vi "Read Unfiltered Debug Data.vi"(8 "error in (no error)":errorcluster, 11 "Debugger In":refnum<class "Debugger.lvclass">) -> (0 "error out":errorcluster, 2 "Data Log":refnum<class "Debug Data.lvclass">[](array[class]), 3 "Debugger Out":refnum<class "Debugger.lvclass">)   [LabVIEW 2020, in "Debugger.lvclass"]
uses:
  Debugger.lvclass
  Debug Data/Debug Data.lvclass
  Debug Log/Debug Log.lvclass/Debug Log.ctl
  Debugger.lvclass/Debugger.ctl
  Debug Log/Debug Log.lvclass
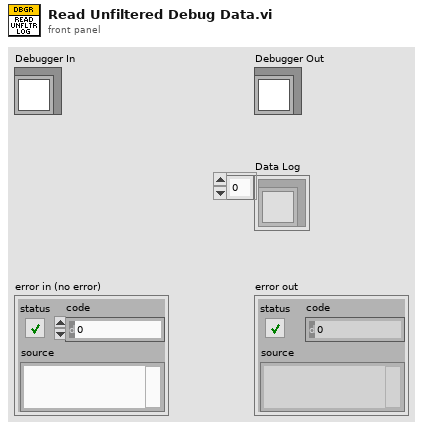
[diagram p1: front panel]
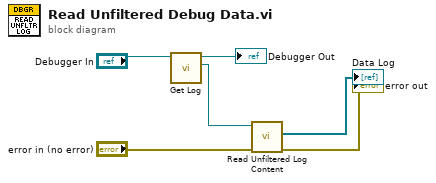
[diagram p0: block diagram]
diagram:
  n1 = call "Get Log.vi"("Debugger in"="Debugger In") -> ("Log"=w1:refnum<class "Debug Log.lvclass">, "Debugger out"=→"Debugger Out":refnum<class "Debugger.lvclass">)  [unwired: 8 in, 1 out]
  n2 = call "Read Unfiltered Log Content.vi"("error in (no error)"="error in (no error)", "Debug Log In"=w1) -> ("error out"=→"error out":errorcluster, "Data Log"=→"Data Log":refnum<class "Debug Data.lvclass">[])  [unwired: 7 in, 1 out]
